vi "SafeParser_Float.vi"(5 "Maximum":dbl, 7 "Minimum":dbl, 9 "Array Index":i32, 11 "String Array":string[](array[string])) -> (0 "Error Out":errorcluster, 3 "Typecast  Value":dbl)   [LabVIEW 2020]
doc: "This VI is configured for polymorphic use and takes in an array of strings and converts one of those strings (specified by an index) to a double. Error checking is performed including checking for acceptable data ranges. This VI is intended for use for the FRC 4265 autonomous parameter strings."
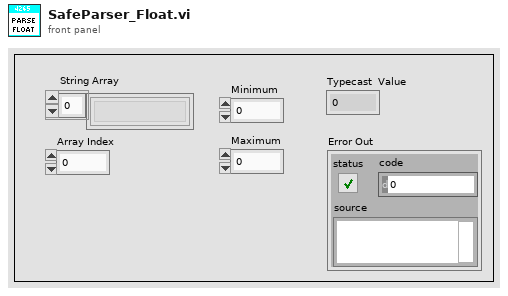
[diagram p1: front panel]
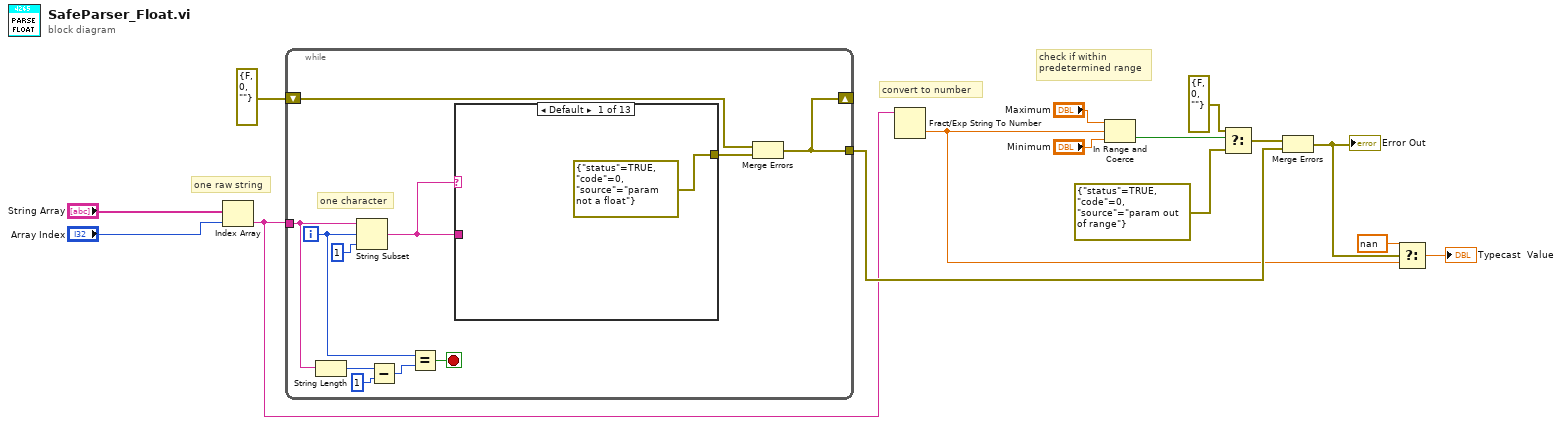
[diagram p0: block diagram]
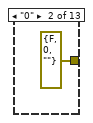
[diagram p2: hidden frame]
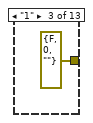
[diagram p3: hidden frame]
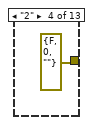
[diagram p4: hidden frame]
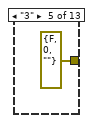
[diagram p5: hidden frame]
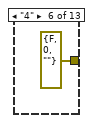
[diagram p6: hidden frame]
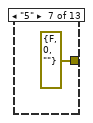
[diagram p7: hidden frame]
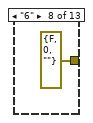
[diagram p8: hidden frame]
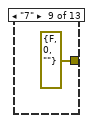
[diagram p9: hidden frame]
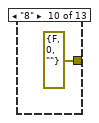
[diagram p10: hidden frame]
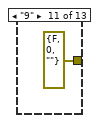
[diagram p11: hidden frame]
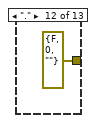
[diagram p12: hidden frame]
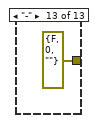
[diagram p13: hidden frame]
diagram:
  # "convert to number"
  # "check if within\npredetermined range"
  # "one raw string"
  n1 = Index Array(array="String Array", index="Array Index") -> (element=w5:string)
  n2 = while {
    tunnel: w5 -> [w25]
    shift-right: [w16] -> _
    shift-left: errorcluster {"status"=FALSE, "code"=0, "source"=""} ("error constant") -> [w17]
    tunnel: [w16] -> w7
    i -> [w22]
    stop <- w24 stop-if-true
    # "one character"
    n3 = String Length(string=w25) -> (length=w21:i32)
    n4 = String Subset(string=w25, offset (0)=w22, length (rest)=1) -> (substring=w23:string)
    n5 = Subtract(x=w21, y=1) -> (x-y=w19:i32)
    n6 = Equal?(x=w22, y=w19) -> (x = y?=w24:bool)
    n7 = case shown="Default" w23 {
      tunnel: w23 -> [_ _ _ _ _ _ _ _ _ _ _ _ _]
      tunnel: [errorcluster {"status"=TRUE, "code"=0, "source"="param not a float"} ("error constant") errorcluster {"status"=FALSE, "code"=0, "source"=""} ("error constant") errorcluster {"status"=FALSE, "code"=0, "source"=""} ("error constant") errorcluster {"status"=FALSE, "code"=0, "source"=""} ("error constant") errorcluster {"status"=FALSE, "code"=0, "source"=""} ("error constant") errorcluster {"status"=FALSE, "code"=0, "source"=""} ("error constant") errorcluster {"status"=FALSE, "code"=0, "source"=""} ("error constant") errorcluster {"status"=FALSE, "code"=0, "source"=""} ("error constant") errorcluster {"status"=FALSE, "code"=0, "source"=""} ("error constant") errorcluster {"status"=FALSE, "code"=0, "source"=""} ("error constant") errorcluster {"status"=FALSE, "code"=0, "source"=""} ("error constant") errorcluster {"status"=FALSE, "code"=0, "source"=""} ("error constant") errorcluster {"status"=FALSE, "code"=0, "source"=""} ("error constant")] -> w18
      frame Default {
      }
      frame "0" {
      }
      frame "1" {
      }
      frame "2" {
      }
      frame "3" {
      }
      frame "4" {
      }
      frame "5" {
      }
      frame "6" {
      }
      frame "7" {
      }
      frame "8" {
      }
      frame "9" {
      }
      frame "." {
      }
      frame "-" {
      }
    }
    n8 = Merge Errors(w17, w18) -> (w16:errorcluster)
  }
  n9 = Fract/Exp String To Number(string=w5) -> (number=w3:dbl)  [unwired: 3 in, 1 out]
  n10 = In Range and Coerce(upper limit="Maximum", x=w3, lower limit="Minimum") -> (In Range?=w11:bool)  [unwired: 1 out]
  n11 = Select(t=errorcluster {"status"=FALSE, "code"=0, "source"=""} ("error constant"), s=w11, f=errorcluster {"status"=TRUE, "code"=0, "source"="param out of range"} ("error constant")) -> (s? t:f=w8:errorcluster)
  n12 = Merge Errors(w8, w7) -> (w4:errorcluster)
  "Error Out" <- w4
  n13 = Select(t=nan, s=w4, f=w3) -> (s? t:f=→"Typecast  Value":dbl)
